vi "CameraConnect.vi"(8 "error in (no error)":errorcluster, 9 "serial":u64 format="%x", 10 "name":string, 11 "AndorSDK2 in":refnum<class "Andor2.lvclass">) -> (0 "error out":errorcluster, 2 "CameraInfo":T1 {"serial" format="%x"}, 3 "AndorSDK2 out":refnum<class "Andor2.lvclass">)   [LabVIEW 2010, in "Andor2.lvclass"]
uses:
  Andor2.lvclass
  CameraBase/CameraInfo.ctl
  Andor2.lvclass/Andor2.ctl
  CameraBase/CameraBase.lvclass
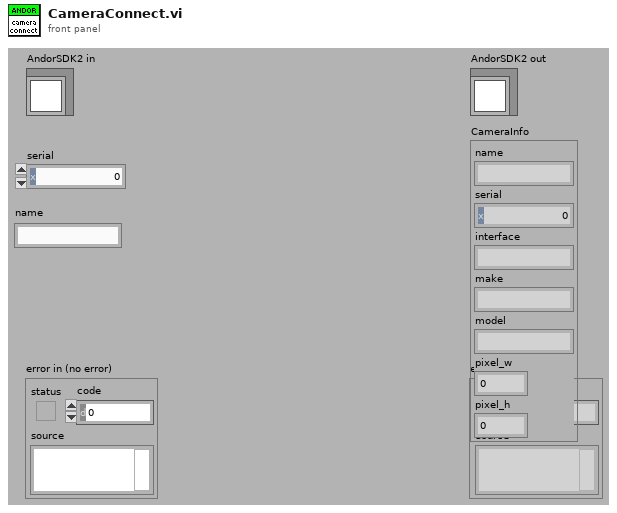
[diagram p1: front panel]
types:
  T1 = typedef "CameraInfo.ctl" = cluster{"name":string, "serial":u64, "interface":string, "make":string, "model":string, "pixel_w":dbl, "pixel_h":dbl}
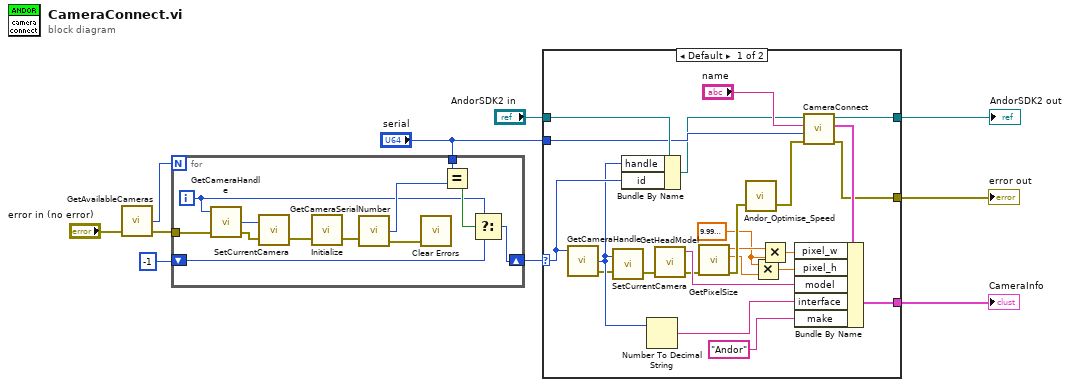
[diagram p0: block diagram]
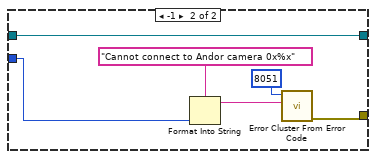
[diagram p2: hidden frame]
diagram:
  n1 = call <userlib>:"GetAvailableCameras.vi"("error in (no error)"="error in (no error)") -> ("error out"=w7:errorcluster, "totalCameras"=w6:i32)  [unwired: 2 in, 1 out]
  n2 = for {
    N: w6 -> [_]
    tunnel: w7 -> [w15]
    shift-right: [w13] -> w2
    shift-left: -1 -> [w14]
    tunnel: "serial" -> [w11]
    i -> [w16]
    n3 = call <userlib>:"GetCameraHandle.vi"("error in (no error)"=w15, "cameraIndex"=w16) -> ("error out"=w18:errorcluster, "cameraHandle"=w22:i32)  [unwired: 1 in, 1 out]
    n4 = call <userlib>:"SetCurrentCamera.vi"("error in (no error)"=w18, "cameraHandle"=w22) -> ("error out"=w19:errorcluster)  [unwired: 1 out]
    n5 = call <userlib>:"Initialize.vi"("error in (no error)"=w19) -> ("error out"=w21:errorcluster)  [unwired: 1 in, 1 out]
    n6 = call <userlib>:"GetCameraSerialNumber.vi"("error in (no error)"=w21) -> ("error out"=w12:errorcluster, "number"=w20:i32)  [unwired: 2 in, 1 out]
    n7 = call <vilib>:"Clear Errors.vi"("error in (no error)"=w12) -> ()  [unwired: 6 in, 1 out]
    n8 = Equal?(x=w11, y=w20) -> (x = y?=w17:bool)
    n9 = Select(t=w16, s=w17, f=w14) -> (s? t:f=w13:i32)
  }
  n10 = case shown="Default" w2 {
    selector: w2 -> [w37 _]
    tunnel: "AndorSDK2 in" -> [w45 w51]
    tunnel: "serial" -> [w44 w46]
    tunnel: [w23 w51] -> w9
    tunnel: [w41 _] -> w8
    tunnel: [w32 w47] -> w1
    frame Default {
      w24 = sgl 1e-06 ("xsize")
      n11 = call <userlib>:"GetCameraHandle.vi"("cameraIndex"=w37) -> ("error out"=w35:errorcluster, "cameraHandle"=w36:i32)  [unwired: 2 in, 1 out]
      n12 = call <userlib>:"SetCurrentCamera.vi"("error in (no error)"=w35, "cameraHandle"=w36) -> ("error out"=w30:errorcluster)  [unwired: 1 out]
      n13 = Bundle By Name(cluster=w45, "handle"=w36, "id"=w37) -> (w40:refnum<class "Andor2.lvclass">)
      n14 = Number To Decimal String(number=w36) -> (decimal integer string=w39:string)  [unwired: 1 in]
      n15 = call <userlib>:"GetHeadModel.vi"("error in (no error)"=w30) -> ("error out"=w31:errorcluster, "model"=w34:string)  [unwired: 2 in, 1 out]
      n16 = call <userlib>:"GetPixelSize.vi"("error in (no error)"=w31) -> ("error out"=w29:errorcluster, "ysize"=w25:sgl, "xsize"=w26:sgl)  [unwired: 3 in, 1 out]
      n17 = call <userlib>:"Andor_Optimise_Speed.vi"("error in"=w29) -> ("error out"=w33:errorcluster)  [unwired: 1 in, 1 out]
      n18 = Multiply(x=w24, y=w25) -> (x*y=w27:sgl)
      n19 = Multiply(x=w26, y=w24) -> (x*y=w28:sgl)
      n20 = call-parent "CameraConnect.vi"("error in (no error)"=w33, "serial"=w44, "name"="name", "CameraBase in"=w40) -> ("error out"=w32:errorcluster, "CameraInfo"=w42:T1, "CameraBase out"=w23:refnum<class "Andor2.lvclass">)  [unwired: 5 in]
      n21 = Bundle By Name(cluster=w42, "pixel_w"=w28, "pixel_h"=w27, "model"=w34, "interface"=w39, "make"="Andor") -> (w41:T1)
    }
    frame -1 {
      n22 = Format Into String(format string="Cannot connect to Andor camera 0x%x", w46) -> (resulting string=w49:string)  [unwired: 2 in, 1 out]
      n23 = call <vilib>:"Error Cluster From Error Code.vi"("error message (\"\")"=w49, "error code (0)"=8051) -> ("error out"=w47:errorcluster)  [unwired: 7 in]
    }
  }
  "error out" <- w1
  "AndorSDK2 out" <- w9
  "CameraInfo" <- w8
